vi "Get Number of Clones.vi"(8 "error in (no error)":errorcluster, 11 "Service in":refnum<class "Service.lvclass">) -> (0 "error out":errorcluster, 3 "Number of Clones":i32)   [LabVIEW 2024, in "Ramses Framework.lvlib" / "Service.lvclass"]
uses:
  Service.lvclass
  Service.lvclass/Service.ctl
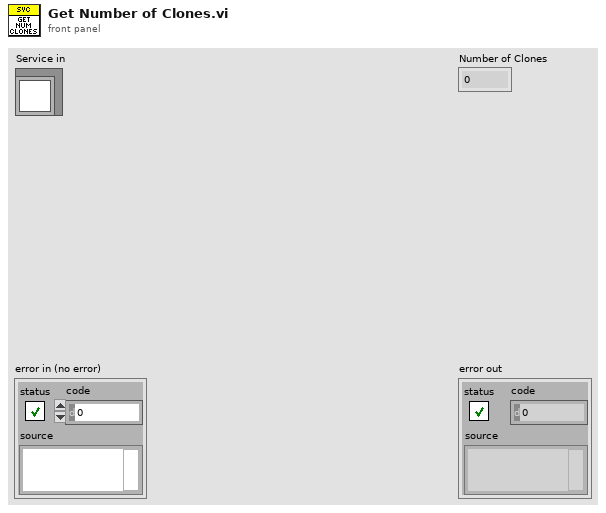
[diagram p1: front panel]
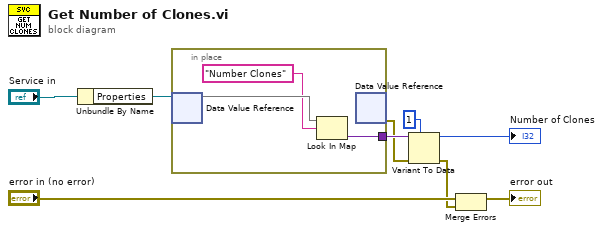
[diagram p0: block diagram]
diagram:
  n1 = Unbundle By Name("Service in") -> ("Properties"=w8:refnum<data-value>)
  n2 = in-place {
    in-place-border: [w10] -> w5
    n3 = in-place-dvr #1(w8) -> (w12:map{string, variant})  [unwired: 1 out]
    n4 = Look In Map(map=w12, key="Number Clones" ("Key")) -> (value=w10:variant)  [unwired: 1 in, 1 out]
    n5 = in-place-dvr #1() -> (w3:errorcluster)  [unwired: 1 in, 1 out]
  }
  n6 = Variant To Data(error in=w3, type=1, Variant=w5) -> (data=→"Number of Clones":i32, error out=w2:errorcluster)
  n7 = Merge Errors("error in (no error)", w2) -> (→"error out":errorcluster)
